vi "DOF Vector Lookup.vi"(10 "DOF Vectors":T1(ring)) -> (1 "IsForce":bool, 2 "Index":u32)   [LabVIEW 2009]
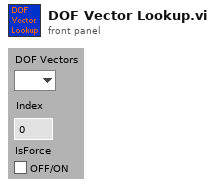
[diagram p1: front panel]
types:
  T1 = enum16{" ", "Dx", "Dy", "Dz", "Rx", "Ry", "Rz", "Fx", "Fy", "Fz", "Mx", "My", "Mz"}
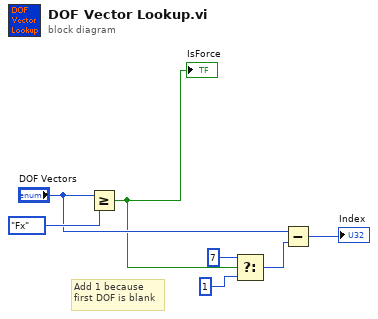
[diagram p0: block diagram]
diagram:
  # "Add 1 because \nfirst DOF is blank"
  n1 = Greater Or Equal?(x="DOF Vectors", y=T1."Fx") -> (x >= y?=w5:bool)
  "IsForce" <- w5
  n2 = Select(t=u32 7, s=w5, f=u32 1) -> (s? t:f=w4:u32)
  n3 = Subtract(x="DOF Vectors", y=w4) -> (x-y=→"Index":u32)
